vi "Runtime test.vi"() -> (0 "input lookup error":errorcluster, 1 "init error":errorcluster, 2 "correct execution settings":bool, 3 "output lookup error":errorcluster, 4 "input error":errorcluster, 5 "serialization problem":errorcluster, 8 "final error":errorcluster, 9 "output error":errorcluster)   [LabVIEW 2014, in "Daqmx Module tests.lvlib"]
doc: "This VI shows an example for how to test the Runtime functionality of the module. This will need to be modified according to module functionality."
uses:
  Daqmx Module tests.lvlib
  module/execution/Daqmx Module runtime.lvclass
  <vilib>/NI/Tag Bus/dictionary/data dictionary.lvclass/data dictionary.ctl
  <vilib>/NI/Tag Bus/dictionary/lookup polymorphs/locate double.vi
  <vilib>/NI/Tag Bus/table/data polymorphs/read many/read Doubles.vi
  <vilib>/NI/Tag Bus/dictionary/search/find data index.vi
  <vilib>/NI/Tag Bus/dictionary/search/search string list.vi
  <vilib>/NI/Tag Bus/dictionary/tag not found.vi
  module/configuration/Daqmx Module configuration.lvclass
  <vilib>/NI/Tag Bus/dictionary/data dictionary.lvclass
  <vilib>/NI/Tag Bus/table/data table.lvlib
  <vilib>/NI/Tag Bus/table/data polymorphs/write one/write Double.vi
panel:
  in  "stop":bool
  out "Waveform Chart":T1(graph)
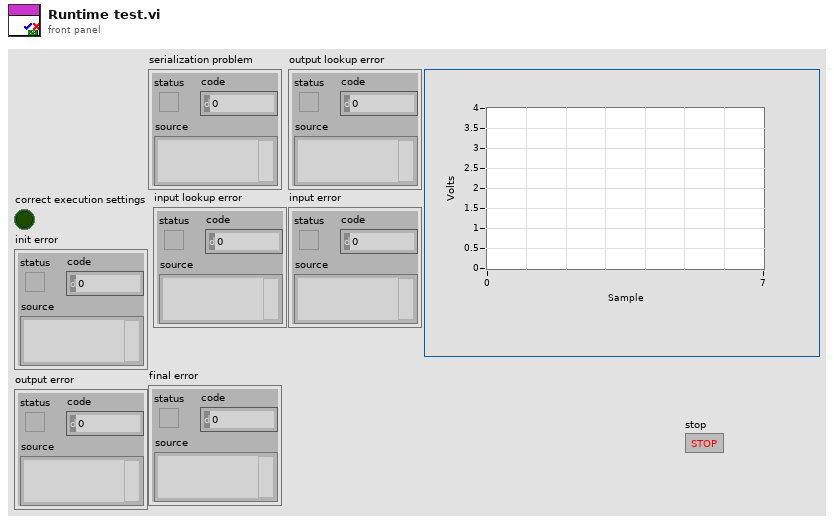
[diagram p1: front panel]
types:
  T1 = cluster{"values[0]":dbl, "values[1]":dbl, "values[2]":dbl, "values[3]":dbl, "values[4]":dbl, "values[5]":dbl, "values[6]":dbl, "values[7]":dbl, "values[8]":dbl}
  T2 = typedef "TBM channel.lvclass/data tables.ctl" = cluster{"input data":T3, "processing parameter":T3, "processing result":T3, "output data":T3}
  T3 = typedef "tag bus.lvlib/dictionary table pair.ctl" = cluster{"data dictionary":refnum<class "data dictionary.lvclass">, "data table":T4}
  T4 = typedef "tag bus.lvlib/data table.lvlib/data table.ctl" = cluster{"Double":dbl[], "Single":sgl[], "I64":i64[], "I32":i32[], "I16":i16[], "I8":i8[], "U64":u64[], "U32":u32[], "U16":u16[], "U8":u8[], "Boolean":bool[], "String":string[], "Array of Double":cluster{"DBL Array":dbl[]}[], "Array of Single":cluster{"SGL Array":sgl[]}[], "Array of I64":cluster{"I64 Array":i64[]}[], "Array of I32":cluster{"I32 Array":i32[]}[], "Array of I16":cluster{"I16 Array":i16[]}[], "Array of I8":cluster{"I8 Array":i8[]}[], "Array of U64":cluster{"U64 Array":u64[]}[], "Array of U32":cluster{"U32 Array":u32[]}[], "Array of U16":cluster{"U16 Array":u16[]}[], "Array of U8":cluster{"U8 Array":u8[]}[], "Array of Boolean":cluster{"Boolean Array":bool[]}[], "Array of String":cluster{"String Array":string[]}[]}
  T5 = typedef "TBM module execution interface.lvclass/execution settings.ctl" = cluster{"reads inputs":bool, "processes data":bool, "writes outputs":bool}
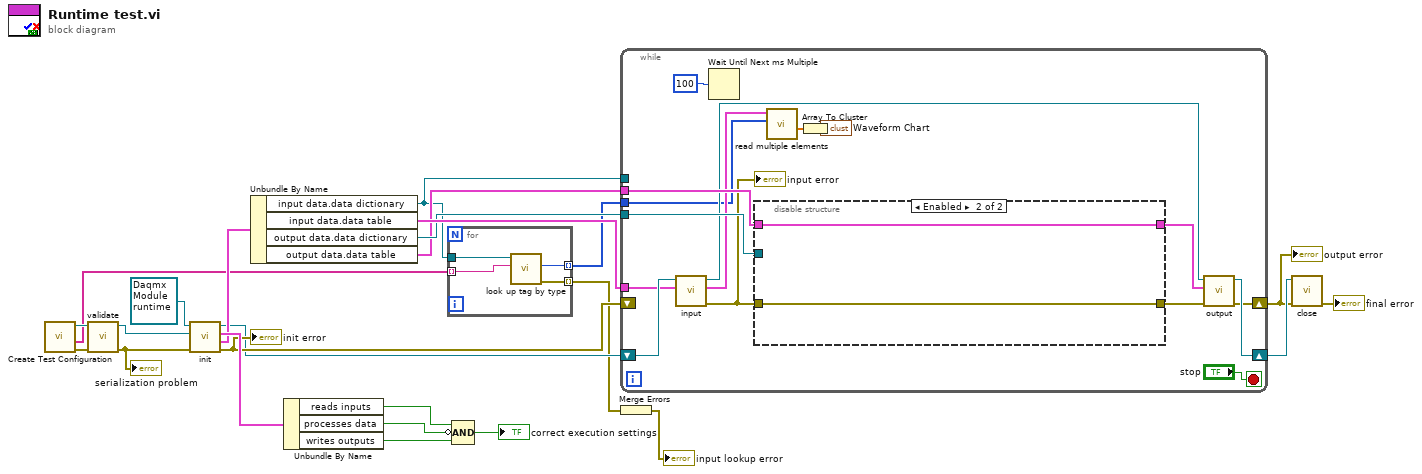
[diagram p0: block diagram]
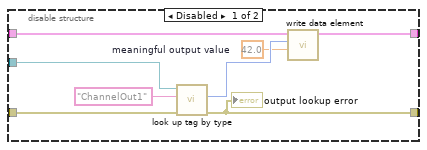
[diagram p2: hidden frame]
diagram:
  n1 = call "Create Test Configuration.vi"() -> ("error out"=w6:errorcluster, "Names"=w4:string[], "Module Configuration"=w7:refnum<class "Daqmx Module configuration.lvclass">)  [unwired: 6 in, 3 out]
  n2 = call-dynamic "validate.vi"("error in"=w6, "Daqmx Module configuration in"=w7) -> ("error out"=w23:errorcluster, "Daqmx Module configuration out"=w22:refnum<class "Daqmx Module configuration.lvclass">)  [unwired: 8 in]
  "serialization problem" <- w23
  n3 = call-dynamic "init.vi"("error in"=w23, "TBM module configuration in"=w22, "Daqmx Module runtime in"=refnum<class "Daqmx Module runtime.lvclass"> refnum ("tag bus configurable plugin module")) -> ("error out"=w15:errorcluster, "data allocations"=w16:T2, "execution settings"=w21:T5, "Daqmx Module runtime out"=w13:refnum<class "Daqmx Module runtime.lvclass">)  [unwired: 5 in]
  "init error" <- w15
  n4 = Unbundle By Name(w16) -> ("input data.data dictionary"=w5:refnum<class "data dictionary.lvclass">, "input data.data table"=w14:T4, "output data.data dictionary"=w12:refnum<class "data dictionary.lvclass">, "output data.data table"=w11:T4)
  n5 = Unbundle By Name(w21) -> ("reads inputs"=w18:bool, "processes data"=w20:bool, "writes outputs"=w19:bool)
  n6 = for {
    tunnel: w5 -> [w28]
    tunnel: w4 -> [w27] mode=indexing
    tunnel: [w26] -> w3 mode=indexing
    tunnel: [w25] -> w2 mode=indexing
    n7 = call-poly <vilib>:"look up tag by type.vi"("name"=w27, "data dictionary in"=w28) -> ("error out"=w25:errorcluster, "index"=w26:i32)  [unwired: 7 in, 1 out]
  }
  n8 = Compound Arithmetic op=AND(w18, invert w20, w19) -> (→"correct execution settings":bool)
  n9 = while {
    tunnel: w5 -> [_]
    tunnel: w14 -> [w33]
    tunnel: w12 -> [w43]
    tunnel: w11 -> [w42]
    shift-right: [w36] -> w9
    shift-left: w15 -> [_]
    shift-right: [w37] -> w10
    shift-left: w13 -> [w44]
    tunnel: w3 -> [w31]
    stop <- "stop" stop-if-true
    n10 = call-dynamic "input.vi"("data table in"=w33, "Daqmx Module runtime in"=w44) -> ("error out"=w41:errorcluster, "data table out"=w32:T4, "Daqmx Module runtime out"=w39:refnum<class "Daqmx Module runtime.lvclass">)  [unwired: 7 in]
    "input error" <- w41
    n11 = Wait Until Next ms Multiple(millisecond multiple=u32 100) -> ()  [unwired: 1 out]
    n12 = disable-structure shown="Enabled" {
      disable-tunnel: w43 -> [w52 _]
      disable-tunnel: w42 -> [w49 w53]
      disable-tunnel: w41 -> [w48 w54]
      disable-tunnel: [w46 w54] -> w40
      disable-tunnel: [w45 w53] -> w38
      frame Disabled {
        w47 = 42.0  # meaningful output value
        n13 = call-poly <vilib>:"look up tag by type.vi"("error in"=w48, "name"="ChannelOut1" ("channel name"), "data dictionary in"=w52) -> ("error out"=w46:errorcluster, "index"=w50:i32)  [unwired: 6 in, 1 out]
        "output lookup error" <- w46
        n14 = call-poly <vilib>:"write data element.vi"("value"=w47, "index"=w50, "data table in"=w49) -> ("data table out"=w45:T4)  [unwired: 8 in]
      }
      frame Enabled {
      }
    }
    n15 = call-poly <vilib>:"read multiple elements.vi"("indices"=w31, "data table in"=w32) -> ("values"=w30:dbl[])  [unwired: 8 in, 1 out]
    n16 = Array To Cluster(array=w30) -> (cluster=→"Waveform Chart":T1)
    n17 = call-dynamic "output.vi"("error in"=w40, "data table in"=w38, "Daqmx Module runtime in"=w39) -> ("error out"=w36:errorcluster, "Daqmx Module runtime out"=w37:refnum<class "Daqmx Module runtime.lvclass">)  [unwired: 6 in, 1 out]
  }
  "output error" <- w9
  n18 = Merge Errors(w2) -> (→"input lookup error":errorcluster)
  n19 = call-dynamic "close.vi"("error in"=w9, "Daqmx Module runtime in"=w10) -> ("error out"=→"final error":errorcluster)  [unwired: 9 in]
